vi "DrawImageWithMaskToPictureGreyscale.vi"(7 "Image Draw Offset (Default 0,0)":T1, 8 "error in (no error)":errorcluster, 10 "Greyscale Mask":refnum<data-value>, 11 "Greyscale Image Source":refnum<data-value>) -> (0 "error out":errorcluster, 3 "Picture":picture)   [LabVIEW 2020, in "g_ar_toolkit.image.lvlib"]
uses:
  g_ar_toolkit.image.lvlib
  Image Draw Offset.ctl
  <vilib>/Utility/error.llb/Error Cluster From Error Code.vi
  9ae995ca-ccda-485c-89ac-02736fde3e8e.vi
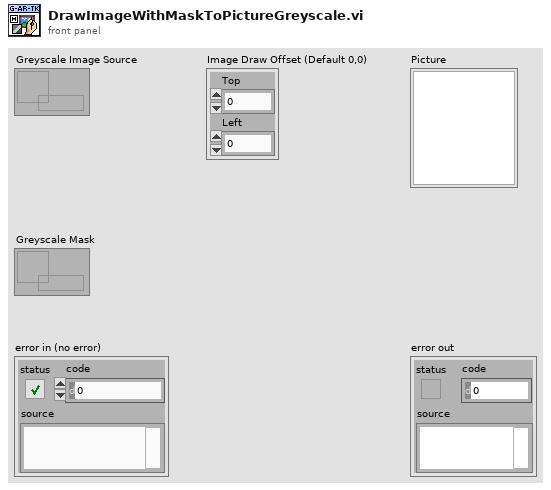
[diagram p1: front panel]
types:
  T1 = typedef "g_ar_toolkit.image.lvlib/Image Draw Offset.ctl" = cluster{"Top":i16, "Left":i16}
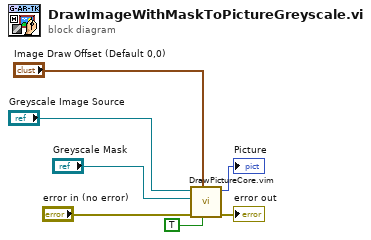
[diagram p0: block diagram]
diagram:
  n1 = call "DrawPictureCore.vim"("HasMask"=TRUE, "Image Draw Offset"="Image Draw Offset (Default 0,0)", "error in (no error)"="error in (no error)", "Image Mask"="Greyscale Mask", "Image Src"="Greyscale Image Source") -> ("error out"=→"error out":errorcluster, "Picture"=→"Picture":picture)  [unwired: 5 in]
